vi "RhodeSchwarz_write_tdms_header.vi"(8 "error in (no error)":errorcluster, 10 "wfm info":T1(array[cluster]), 11 "Refnum in":refnum<k34>) -> (0 "error out":errorcluster, 3 "Refnum out":refnum<k34>)   [LabVIEW 2020, in "RohdeSchwarz_RTA4000.lvclass"]
uses:
  RohdeSchwarz_RTA4000.lvclass
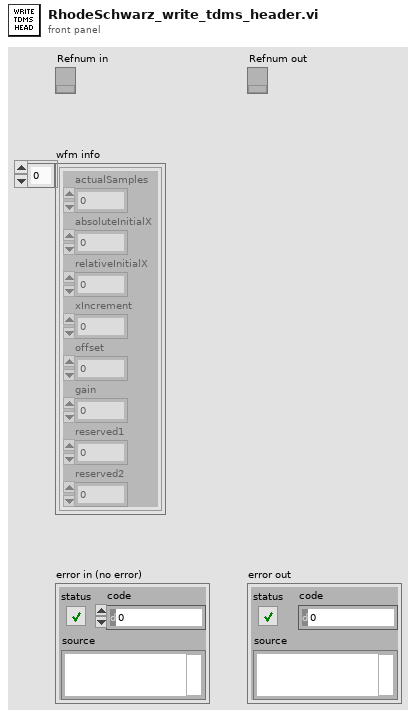
[diagram p1: front panel]
types:
  T1 = cluster{"actualSamples":i32, "absoluteInitialX":dbl, "relativeInitialX":dbl, "xIncrement":dbl, "offset":dbl, "gain":dbl, "reserved1":dbl, "reserved2":dbl}[]
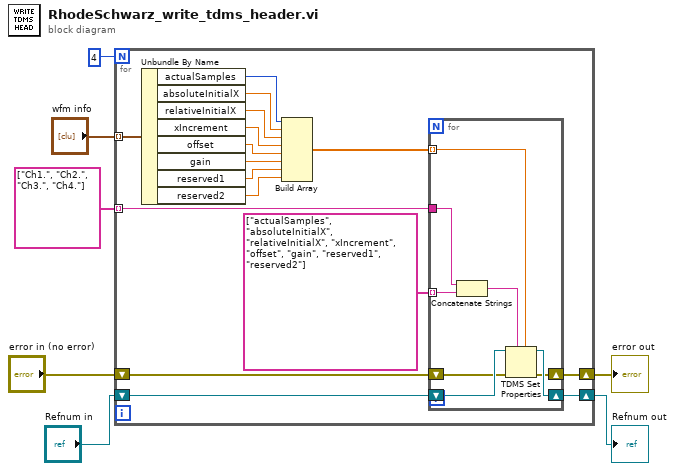
[diagram p0: block diagram]
diagram:
  n1 = for {
    N: 4 -> [_]
    tunnel: "wfm info" -> [w23] mode=indexing
    shift-right: [w11] -> w5
    shift-left: "Refnum in" -> [w12]
    shift-right: [w9] -> w7
    shift-left: "error in (no error)" -> [w10]
    tunnel: string[] ["Ch1.", "Ch2.", "Ch3.", "Ch4."] -> [w8] mode=indexing
    n2 = Unbundle By Name(w23) -> ("actualSamples"=w22:i32, "absoluteInitialX"=w21:dbl, "relativeInitialX"=w20:dbl, "xIncrement"=w19:dbl, "offset"=w18:dbl, "gain"=w17:dbl, "reserved1"=w16:dbl, "reserved2"=w15:dbl)
    n3 = Build Array(w22, w21, w20, w19, w18, w17, w16, w15) -> (w14:dbl[])
    n4 = for {
      tunnel: w14 -> [w24] mode=indexing
      tunnel: string[] ["actualSamples", "absoluteInitialX", "relativeInitialX", "xIncrement", "offset", "gain", "reserved1", "reserved2"] -> [w27] mode=indexing
      shift-right: [w30] -> w11
      shift-left: w12 -> [w31]
      shift-right: [w28] -> w9
      shift-left: w10 -> [w29]
      tunnel: w8 -> [w26]
      n5 = Concatenate Strings(w26, w27) -> (w25:string)
      n6 = TDMS Set Properties(5:w24, 7:w25, 8:w29, 11:w31) -> (0:w28:errorcluster, 3:w30:refnum<k34>)  [unwired: 2 in, 2 out]
    }
  }
  "error out" <- w7
  "Refnum out" <- w5
